vi "Begin.vi"(8 "error in":errorcluster) -> (0 "error out":errorcluster)   [LabVIEW 2016]
doc: "Called before other user functions, this VI is expected to open initial I/O refnums, load in file data, and do all program initialization. Notice that the <B>error out</B> terminal is simply used for data flow. Wiring it to other structures or subVIs ensures that this VI runs first."
uses:
  <vilib>/Rock Robotics/WPI/DriverStation/WPI_DriverStationRobotMode2.ctl
  <vilib>/Rock Robotics/WPI/Joystick/WPI_JoystickDeviceEnum.ctl
  <vilib>/Rock Robotics/WPI/ThirdParty/CanMotor/TalonSRX/WPI_CANTalonSRX_APIControlMode.ctl
  <vilib>/Rock Robotics/WPI/SafetyOutput/WPI_SafetyOutputConfigMenu.ctl
  <vilib>/Rock Robotics/SystemInterfaces/DIO/FPGA_DIOPWMChannel.ctl
  <vilib>/Rock Robotics/SystemInterfaces/DIO/FPGA_DIOChannel.ctl
  Robot Global Data.vi
  <vilib>/Rock Robotics/Network Tables/NT Write String Array.vi
  <vilib>/Rock Robotics/WPI/MotorControl/WPI_MotorControlOpen TalonSRX.vi
  <vilib>/Rock Robotics/WPI/MotorControl/WPI_MotorControlOpen Talon.vi
  <vilib>/Rock Robotics/WPI/RobotDrive/WPI_RobotDriveOpen4MotorWithExistingMotors.vi
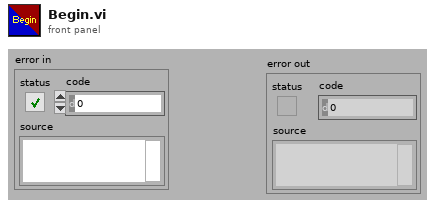
[diagram p1: front panel]
types:
  T1 = typedef "WPI_CANTalonSRX_APIControlMode.ctl" = enum8{"Percent VBus", "Speed", "Position", "Slave", "Unchanged / Invalid", "Voltage Compensation", "Current", "Motion Profile", "Motion Magic"}
  T2 = typedef "FPGA_DIOPWMChannel.ctl" = enum8{"PWM 0", "PWM 1", "PWM 2", "PWM 3", "PWM 4", "PWM 5", "PWM 6", "PWM 7", "PWM 8", "PWM 9", "PWM MXP 0", "PWM MXP 1", "PWM MXP 2", "PWM MXP 3", "PWM MXP 4", "PWM MXP 5", "PWM MXP 6", "PWM MXP 7", "PWM MXP 8", "PWM MXP 9", "Invalid"}
  T3 = typedef "FPGA_DIOChannel.ctl" = enum8{"DIO 0", "DIO 1", "DIO 2", "DIO 3", "DIO 4", "DIO 5", "DIO 6", "DIO 7", "DIO 8", "DIO 9", "DIO MXP 0", "DIO MXP 1", "DIO MXP 2", "DIO MXP 3", "DIO MXP 4", "DIO MXP 5", "DIO MXP 6", "DIO MXP 7", "DIO MXP 8", "DIO MXP 9", "DIO MXP 10", "DIO MXP 11", "DIO MXP 12", "DIO MXP 13", "DIO MXP 14", "DIO MXP 15", "SPI Port CS1", "SPI Port CS2", "SPI Port CS3", "SPI Port MISO", "SPI Port MOSI", "Invalid"}
  T4 = typedef "WPI_JoystickDeviceEnum.ctl" = enum16{"USB 0", "USB 1", "USB 2", "USB 3", "USB 4", "USB 5"}
  T5 = typedef "WPI_SafetyOutputConfigMenu.ctl" = enum16{"Enable", "Disable"}
  T6 = typedef "WPI_DriverStationRobotMode2.ctl" = enum16{"Autonomous Disabled", "Autonomous Enabled", "Teleop Disabled", "Teleop Enabled", "Disconnected", "Finish", "Test Disabled", "Test Enabled", "Emergency Stopped"}
  T7 = typedef "WPI_MotorControlDeviceRef.ctl" = cluster{"DeviceStatus":errorcluster, "Type":T8, "PWM":cluster{"PWM Channel":T2, "DeadBand":T9}, "CAN":cluster{"Device Number":u8, "SetOutput VI Ref":variant, "GetOutput VI Ref":variant, "Enable VI Ref":variant, "Disable VI Ref":variant, "Data":variant}, "Invert":bool}
  T8 = typedef "WPI_MotorControlType.ctl" = enum16{"PWM", "CAN"}
  T9 = typedef "WPI_PWMDeadband.ctl" = cluster{"Name":string, "maxPositivePwm":i32, "minPositivePwm":i32, "centerPwm":i32, "maxNegativePwm":i32, "minNegativePwm":i32, "angularRange":u16}
  T10 = typedef "WPI_JoystickDevRef.ctl" = cluster{"Device":T4}
  T11 = typedef "WPI_DigitalInputDevRef.ctl" = cluster{"DevStatus":errorcluster, "DIO Channel":T3}
  T12 = typedef "WPI_RobotDriveDevRef.ctl" = cluster{"DevStatus":errorcluster, "Motors[]":T7[], "Square Inputs":bool, "Max Output":dbl}
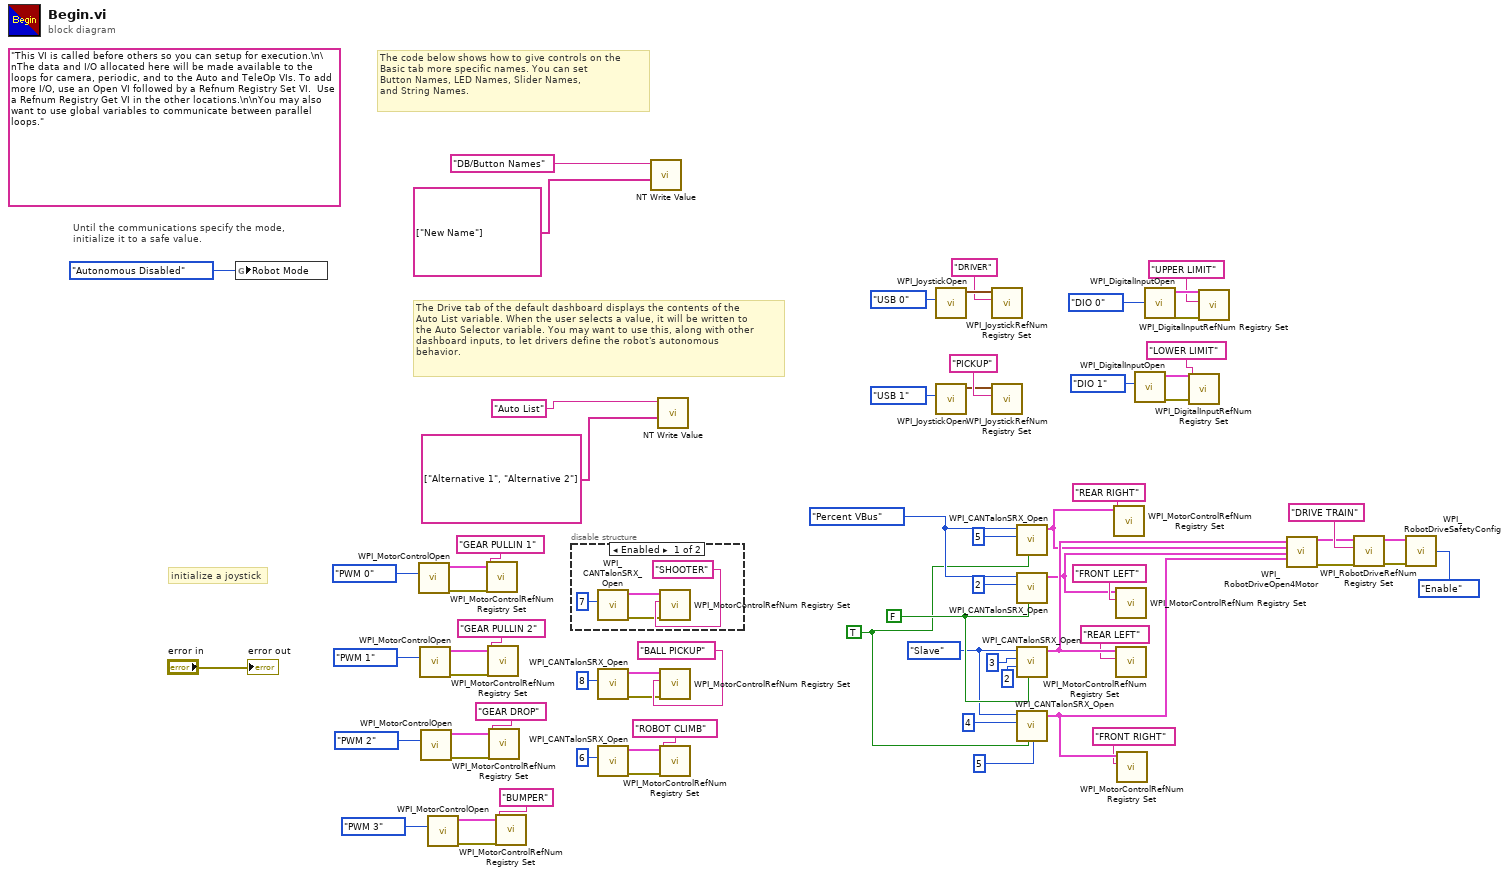
[diagram p0: block diagram]
diagram:
  w16 = WPI_CANTalonSRX_APIControlMode."Slave" ("Control Mode")
  w50 = TRUE ("Invert")
  w51 = FALSE ("Invert")
  w55 = WPI_CANTalonSRX_APIControlMode."Percent VBus" ("Control Mode")
  (unwired) "This VI is called before others so you can setup for execution.\n\nThe data and I/O allocated here will be made available to the loops for camera, periodic, and to the Auto and TeleOp VIs. To add more I/O, use an Open VI followed by a Refnum Registry Set VI.  Use a Refnum Registry Get VI in the other locations.\n\nYou may also want to use global variables to communicate between parallel loops."
  # "The Drive tab of the default dashboard displays the contents of the\nAuto List variable. When the user selects a value, it will be written to\nthe Auto Selector variable. You may want to use this, along with other\ndashboard inputs, to let drivers define the robot's autonomous\nbehavior."
  # "The code below shows how to give controls on the\nBasic tab more specific names. You can set\nButton Names, LED Names, Slider Names,\nand String Names."
  # "initialize a joystick"
  # "Until the communications specify the mode,\ninitialize it to a safe value."
  n1 = global write "Robot Global Data.vi" "Robot Mode"(WPI_DriverStationRobotMode2."Autonomous Disabled" ("Robot Mode")) -> ()
  n2 = call-poly <vilib>:"WPI_MotorControlOpen.vi"("PWM Channel"=FPGA_DIOPWMChannel."PWM 0") -> ("error out"=w3:errorcluster, "MotorControlDeviceRef"=w36:T7)  [unwired: 9 in]
  n3 = call-poly <vilib>:"WPI_MotorControlOpen.vi"("PWM Channel"=FPGA_DIOPWMChannel."PWM 1") -> ("error out"=w4:errorcluster, "MotorControlDeviceRef"=w35:T7)  [unwired: 9 in]
  n4 = call-poly <vilib>:"WPI_MotorControlOpen.vi"("PWM Channel"=FPGA_DIOPWMChannel."PWM 2") -> ("error out"=w2:errorcluster, "MotorControlDeviceRef"=w30:T7)  [unwired: 9 in]
  n5 = call-poly <vilib>:"WPI_MotorControlOpen.vi"("PWM Channel"=FPGA_DIOPWMChannel."PWM 3") -> ("error out"=w1:errorcluster, "MotorControlDeviceRef"=w19:T7)  [unwired: 9 in]
  n6 = call <vilib>:"WPI_MotorControlRefNum Registry Set.vi"("error in (no error)"=w3, "refnum name"="GEAR PULLIN 1", "MotorControlDevRef"=w36) -> ()  [unwired: 7 in, 2 out]
  n7 = call <vilib>:"WPI_MotorControlRefNum Registry Set.vi"("error in (no error)"=w4, "refnum name"="GEAR PULLIN 2", "MotorControlDevRef"=w35) -> ()  [unwired: 7 in, 2 out]
  n8 = call <vilib>:"WPI_MotorControlRefNum Registry Set.vi"("error in (no error)"=w2, "refnum name"="GEAR DROP", "MotorControlDevRef"=w30) -> ()  [unwired: 7 in, 2 out]
  n9 = call <vilib>:"WPI_MotorControlRefNum Registry Set.vi"("error in (no error)"=w1, "refnum name"="BUMPER", "MotorControlDevRef"=w19) -> ()  [unwired: 7 in, 2 out]
  n10 = disable-structure shown="Enabled" {
    frame Enabled {
      n11 = call <vilib>:"WPI_CANTalonSRX_Open.vi"("Device Number"=u8 7) -> ("error out"=w69:errorcluster, "CAN Talon SRX Ref"=w71:T7)  [unwired: 9 in]
      n12 = call <vilib>:"WPI_MotorControlRefNum Registry Set.vi"("error in (no error)"=w69, "refnum name"="SHOOTER", "MotorControlDevRef"=w71) -> ()  [unwired: 7 in, 2 out]
    }
    frame Disabled {
    }
  }
  n13 = call <vilib>:"WPI_CANTalonSRX_Open.vi"("Device Number"=u8 8) -> ("error out"=w6:errorcluster, "CAN Talon SRX Ref"=w44:T7)  [unwired: 9 in]
  n14 = call <vilib>:"WPI_CANTalonSRX_Open.vi"("Device Number"=u8 6) -> ("error out"=w5:errorcluster, "CAN Talon SRX Ref"=w41:T7)  [unwired: 9 in]
  n15 = call-poly <vilib>:"NT Write Value.vi"("String Array"=string[] ["New Name"], "Name"="DB/Button Names") -> ()  [unwired: 9 in, 1 out]
  n16 = call-poly <vilib>:"NT Write Value.vi"("String Array"=string[] ["Alternative 1", "Alternative 2"], "Name"="Auto List") -> ()  [unwired: 9 in, 1 out]
  n17 = call <vilib>:"WPI_MotorControlRefNum Registry Set.vi"("error in (no error)"=w6, "refnum name"="BALL PICKUP", "MotorControlDevRef"=w44) -> ()  [unwired: 7 in, 2 out]
  n18 = call <vilib>:"WPI_MotorControlRefNum Registry Set.vi"("error in (no error)"=w5, "refnum name"="ROBOT CLIMB", "MotorControlDevRef"=w41) -> ()  [unwired: 7 in, 2 out]
  n19 = call <vilib>:"WPI_JoystickOpen.vi"("JoystickDevice"=WPI_JoystickDeviceEnum."USB 0") -> ("JoystickDevRef"=w47:T10)  [unwired: 10 in]
  n20 = call <vilib>:"WPI_JoystickOpen.vi"("JoystickDevice"=WPI_JoystickDeviceEnum."USB 1") -> ("JoystickDevRef"=w66:T10)  [unwired: 10 in]
  n21 = call <vilib>:"WPI_JoystickRefNum Registry Set.vi"("refnum name"="DRIVER", "JoystickDevRef"=w47) -> ()  [unwired: 8 in, 2 out]
  n22 = call <vilib>:"WPI_JoystickRefNum Registry Set.vi"("refnum name"="PICKUP", "JoystickDevRef"=w66) -> ()  [unwired: 8 in, 2 out]
  n23 = call <vilib>:"WPI_CANTalonSRX_Open.vi"("Invert"=w50, "Device Number"=u8 5, "Control Mode"=w55) -> ("CAN Talon SRX Ref"=w13:T7)  [unwired: 7 in, 1 out]
  n24 = call <vilib>:"WPI_CANTalonSRX_Open.vi"("Invert"=w51, "Device Number"=u8 2, "Control Mode"=w55) -> ("CAN Talon SRX Ref"=w12:T7)  [unwired: 7 in, 1 out]
  n25 = call <vilib>:"WPI_CANTalonSRX_Open.vi"("Invert"=w51, "Master Device Number"=u8 2, "Device Number"=u8 3, "Control Mode"=w16) -> ("CAN Talon SRX Ref"=w28:T7)  [unwired: 6 in, 1 out]
  n26 = call <vilib>:"WPI_CANTalonSRX_Open.vi"("Invert"=w50, "Master Device Number"=u8 5, "Device Number"=u8 4, "Control Mode"=w16) -> ("CAN Talon SRX Ref"=w29:T7)  [unwired: 6 in, 1 out]
  n27 = call <vilib>:"WPI_MotorControlRefNum Registry Set.vi"("refnum name"="REAR RIGHT", "MotorControlDevRef"=w13) -> ()  [unwired: 8 in, 2 out]
  n28 = call <vilib>:"WPI_MotorControlRefNum Registry Set.vi"("refnum name"="FRONT LEFT", "MotorControlDevRef"=w12) -> ()  [unwired: 8 in, 2 out]
  n29 = call <vilib>:"WPI_MotorControlRefNum Registry Set.vi"("refnum name"="REAR LEFT", "MotorControlDevRef"=w28) -> ()  [unwired: 8 in, 2 out]
  n30 = call <vilib>:"WPI_MotorControlRefNum Registry Set.vi"("refnum name"="FRONT RIGHT", "MotorControlDevRef"=w29) -> ()  [unwired: 8 in, 2 out]
  n31 = call <vilib>:"WPI_DigitalInputOpen.vi"("DIO Channel"=FPGA_DIOChannel."DIO 1") -> ("error out"=w20:errorcluster, "DigitalInputDevRef"=w21:T11)  [unwired: 9 in]
  n32 = call <vilib>:"WPI_DigitalInputOpen.vi"("DIO Channel"=FPGA_DIOChannel."DIO 0") -> ("error out"=w8:errorcluster, "DigitalInputDevRef"=w11:T11)  [unwired: 9 in]
  n33 = call <vilib>:"WPI_DigitalInputRefNum Registry Set.vi"("error in (no error)"=w20, "refnum name"="LOWER LIMIT", "DigitalInputDevRef"=w21) -> ()  [unwired: 7 in, 2 out]
  n34 = call <vilib>:"WPI_DigitalInputRefNum Registry Set.vi"("error in (no error)"=w8, "refnum name"="UPPER LIMIT", "DigitalInputDevRef"=w11) -> ()  [unwired: 7 in, 2 out]
  n35 = call-poly <vilib>:"WPI_RobotDriveOpen4Motor.vi"("Rear Left Motor Dev Ref"=w28, "Rear Right Motor Dev Ref"=w13, "Front Left Motor Dev Ref"=w12, "Front Right Motor Dev Ref"=w29) -> ("RobotDriveDevRef"=w49:T12, "error out"=w45:errorcluster)  [unwired: 10 in]
  n36 = call <vilib>:"WPI_RobotDriveRefNum Registry Set.vi"("error in (no error)"=w45, "refnum name"="DRIVE TRAIN", "RobotDriveDevRef"=w49) -> ("error out"=w7:errorcluster, "RobotDriveDevRef"=w53:T12)  [unwired: 1 in, 6 out]
  n37 = call <vilib>:"WPI_RobotDriveSafetyConfig.vi"("error in (no error)"=w7, "mode"=WPI_SafetyOutputConfigMenu."Enable", "RobotDriveDevRef"=w53) -> ()  [unwired: 7 in, 2 out]
  "error out" <- "error in"
